vi "Schreiben_verknuepfen_Zahl.vi"(8 "error in (no error)":errorcluster caption="Fehler (Eingang, kein Fehler)", 10 "Order":string, 11 "Zahl":dbl) -> (0 "error out":errorcluster caption="Fehler (Ausgang)", 3 "Verknüpfter String":string)   [LabVIEW 2020, in "Linearisierung v2.lvlib" / "Gasteiler.lvlib" / "HovaCAL_Interface.lvlib" / "KGN.lvlib"]
uses:
  KGN.lvlib
panel:
  in  "Zieladresse":string="FF"
  in  "Quelladresse":string="00"
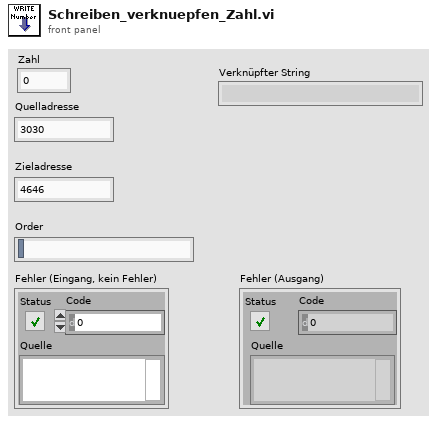
[diagram p1: front panel]
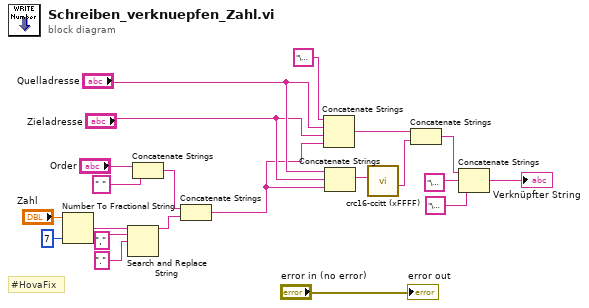
[diagram p0: block diagram]
diagram:
  # "#HovaFix"
  n1 = Number To Fractional String(number="Zahl", precision (6)=i16 7 ("Genauigkeit (6)")) -> (F-format string=w9:string)  [unwired: 2 in]
  n2 = Search and Replace String(input string=w9, search string="," ("Such-String"), replace string="." ("Ersetzungs-String (\"\")")) -> (result string=w6:string)  [unwired: 5 in, 3 out]
  n3 = Concatenate Strings("Order", " " ("String")) -> (w4:string)
  n4 = Concatenate Strings(w4, w6) -> (w5:string)
  n5 = Concatenate Strings("\u0002", "Quelladresse", "Zieladresse", w5) -> (w15:string)
  n6 = Concatenate Strings("Quelladresse", "Zieladresse", w5) -> (w13:string)
  n7 = call "crc16-ccitt (xFFFF).vi"("Message"=w13) -> ("Hex-Integer-String"=w12:string)  [unwired: 8 in, 2 out]
  n8 = Concatenate Strings(w15, w12) -> (w18:string)
  n9 = Concatenate Strings(w18, "\u0003", "\u0006" ("String")) -> (→"Verknüpfter String":string)
  "error out" <- "error in (no error)"
